vi "PITerm.vi"(0 "System no.":i32=1 min=1 max=4 step=1, 1 "String to Send":string) -> (14 "Comm Window":string)   [LabVIEW 2014]
doc: "Simple Terminal Application.\n\nThis vi can be executed in parallel to any existing PI LabVIEW application. \nPlease run XXX_Configuration_Setup.vi and adjust the System no. on the frontpanel to communicate with your PI device.\n\nShorcut keys:\nReturn: Send\nF5: ERR? (with error translation)\nF12: Additional receive function\nPage Up: History up\nPage down: History down"
panel:
  in  "F5":bool
  in  "Command History":string[](array[string])
  in  "Receive":bool
  out "History length":i32
  in  "History DOWN":bool
  in  "History Index":i32
  in  "History UP":bool
  in  "Send":bool
  in  "Clear":bool
  in  "stop":bool
  # "PITerminal"
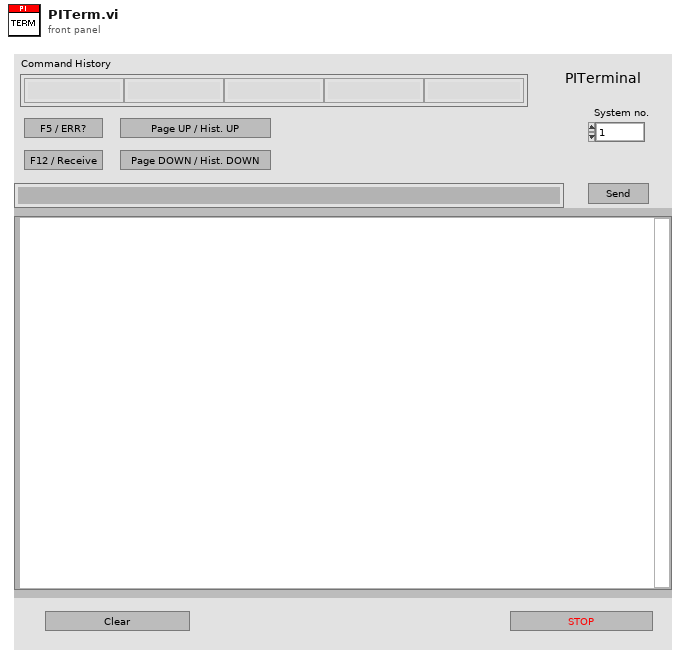
[diagram p1: front panel]
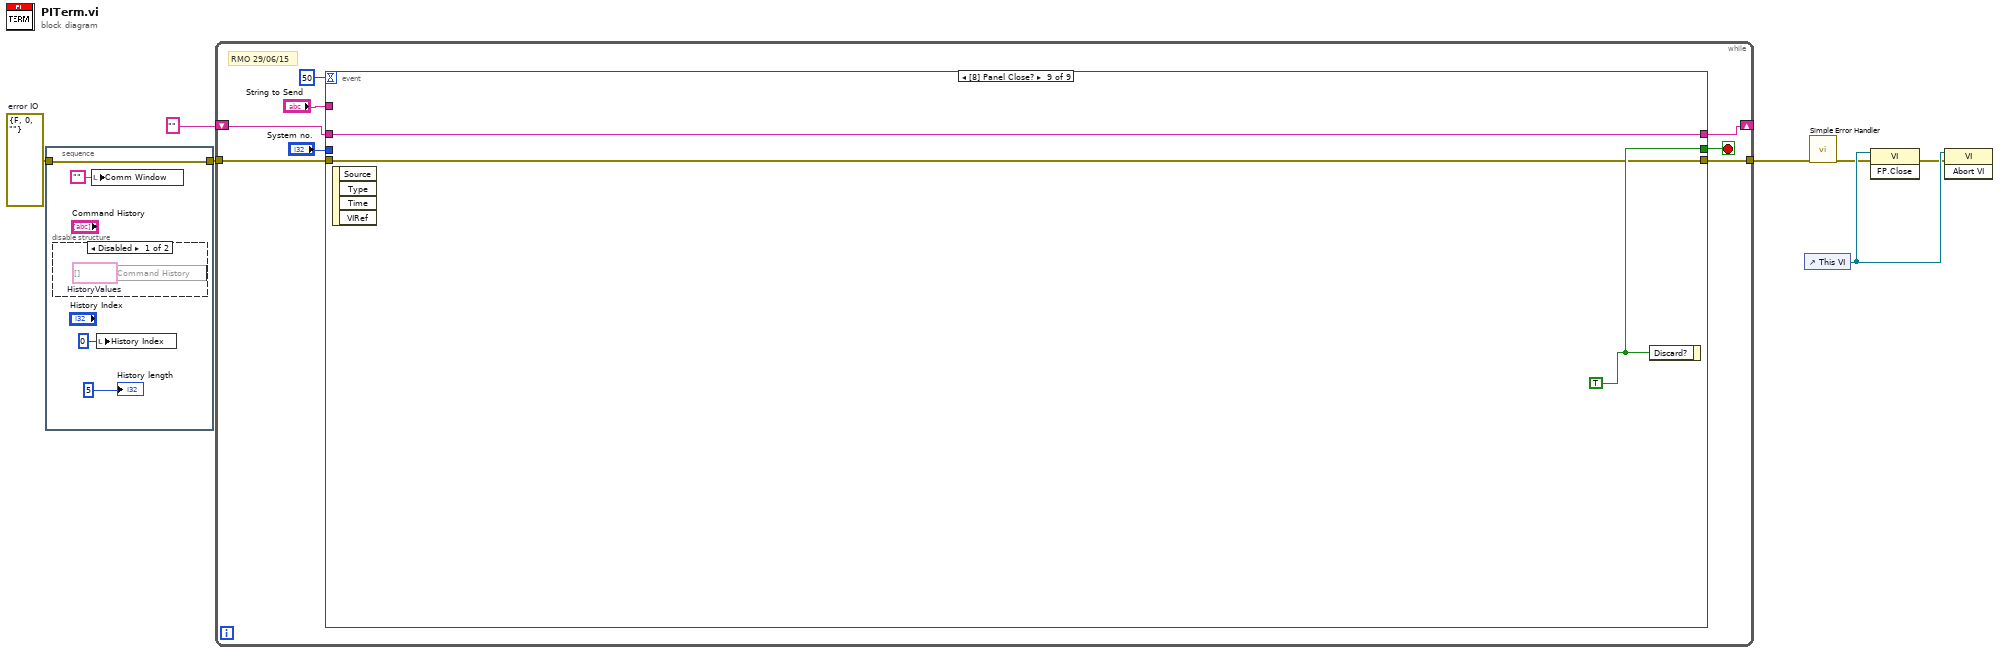
[diagram p0: block diagram]
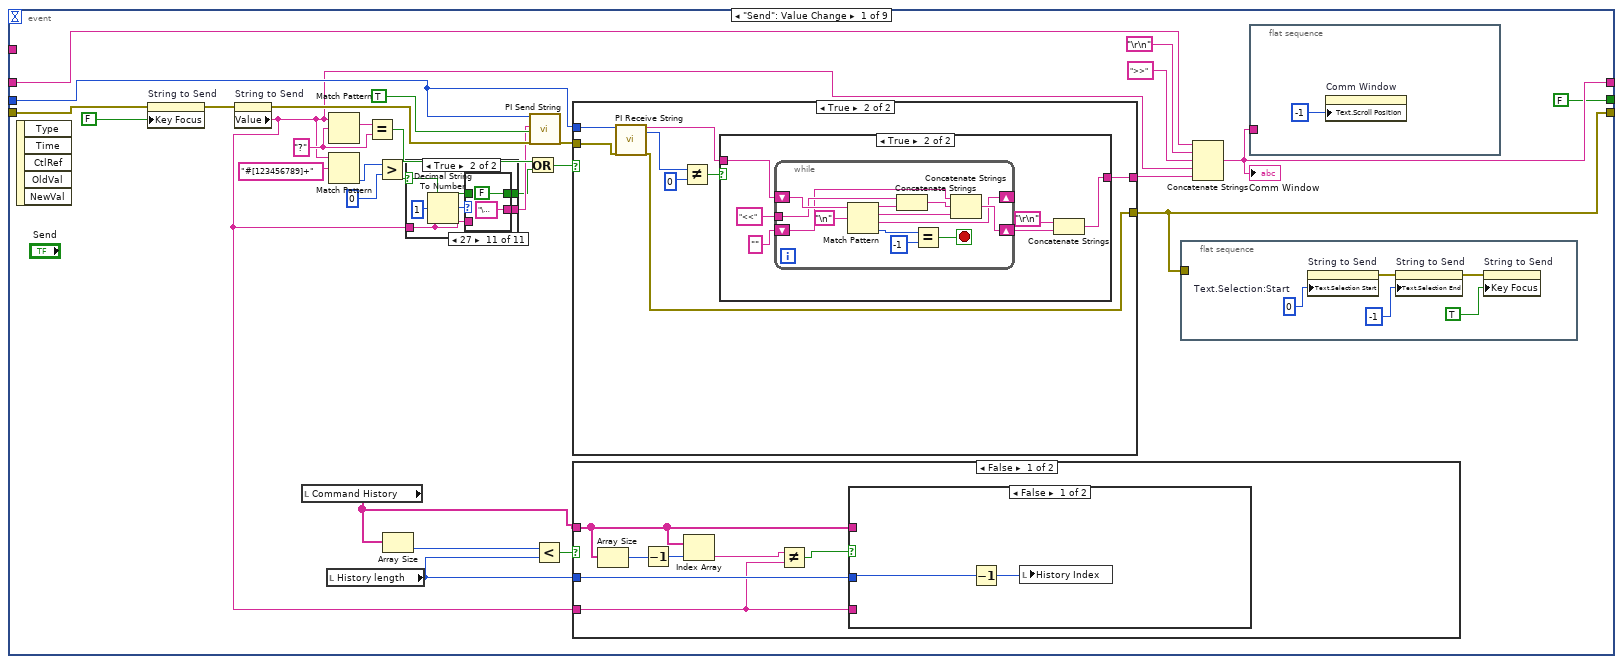
[diagram p3: hidden frame]
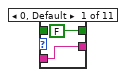
[diagram p5: hidden frame]
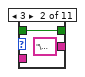
[diagram p6: hidden frame]
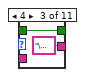
[diagram p7: hidden frame]
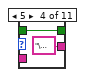
[diagram p8: hidden frame]
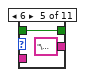
[diagram p9: hidden frame]
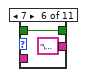
[diagram p10: hidden frame]
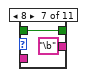
[diagram p11: hidden frame]
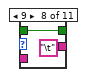
[diagram p12: hidden frame]
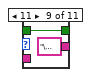
[diagram p13: hidden frame]
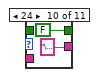
[diagram p14: hidden frame]
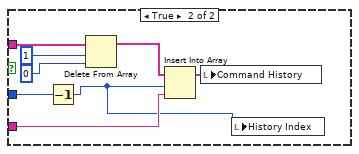
[diagram p15: hidden frame]
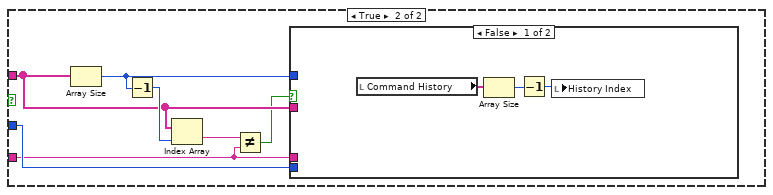
[diagram p16: hidden frame]
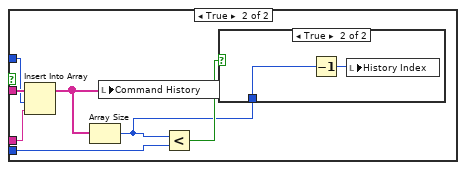
[diagram p17: hidden frame]
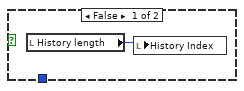
[diagram p18: hidden frame]
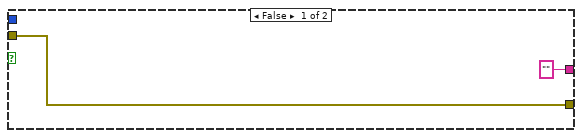
[diagram p19: hidden frame]
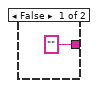
[diagram p20: hidden frame]
diagram:
  w6 = errorcluster {"status"=FALSE, "code"=0, "source"=""}  # error IO
  n1 = stacked-sequence {
    tunnel: w6 -> [w10]
    tunnel: [w10] -> w5
    frame #0 {
      n2 = disable-structure shown="Disabled" {
        frame Disabled {
          w12 = string[] []  # HistoryValues
          n3 = local write "Command History"(w12) -> ()
        }
        frame Enabled {
        }
      }
      n4 = local write "Comm Window"("") -> ()
      n5 = local write "History Index"(0) -> ()
      "History length" <- 5
    }
  }
  n6 = while {
    tunnel: [w19] -> w4
    tunnel: w5 -> [w17]
    shift-right: [w16] -> _
    shift-left: "" -> [w13]
    stop <- w15 stop-if-true
    # "RMO 29/06/15"
    n7 = event shown="[8] Panel Close?" {
      selector: _ -> [_ _ _ _ _ _ _ _ _]
      dyn-events: _ -> [_ _ _ _ _ _ _ _ _]
      timeout: 50 -> [_ _ _ _ _ _ _ _ _]
      tunnel: "String to Send" -> [_ _ _ _ _ _ _ _ _]
      tunnel: [w37 w154 w201 w223 w232 w254 w261 w264 w266] -> w16
      tunnel: [w22 w152 w196 w217 w227 w250 w260 w263 w265] -> w19
      tunnel: "System no." -> [w48 w156 w198 _ _ _ _ _ _]
      tunnel: w17 -> [w36 w157 w199 w216 w227 w250 w260 w263 w265]
      tunnel: [FALSE FALSE FALSE FALSE FALSE FALSE FALSE "stop" w267] -> w15
      tunnel: w13 -> [w47 w155 w200 _ w232 w254 w261 w264 w266]
      event "Send": Value Change {
        w40 = "?"
        n8 = event-data() -> ()  [unwired: 6 out]
        n9 = property on="String to Send" class="Str"(error in=w36, "Key Focus"=FALSE) -> (error out=w34:errorcluster)  [unwired: 1 in, 1 out]
        n10 = property on="String to Send" class="Str"(error in=w34) -> (error out=w33:errorcluster, "Value"=w26:string)  [unwired: 1 in, 1 out]
        n11 = local read "Command History"() -> (w30:string[])
        n12 = local read "History length"() -> (w29:i32)
        n13 = Match Pattern(string=w26, regular expression=w40) -> (match substring=w42:string)  [unwired: 4 out]
        n14 = Match Pattern(string=w26, regular expression="#[123456789]+") -> (offset past match=w28:i32)  [unwired: 4 out]
        n15 = Equal?(x=w42, y=w40) -> (x = y?=w39:bool)
        n16 = Greater?(x=w28, y=0) -> (0:w24:bool)
        n17 = Array Size(array=w30) -> (size(s)=w32:i32)
        n18 = case shown="True" w24 {
          selector: w24 -> [w55 w58]
          tunnel: w26 -> [w56 w59]
          tunnel: [w56 w60] -> w25
          tunnel: [w55 w57] -> w21
          frame False {
          }
          frame True {
            n19 = Decimal String To Number(string=w59, offset=1) -> (number=w61:i32)  [unwired: 2 out]
            n20 = case shown="27" w61 {
              tunnel: [w64 "\u0003" "\u0004" "\u0005" "\u0006" "\u0007" "\b" "\t" "\u000b" "\u0018" "\u001b"] -> w60
              tunnel: w59 -> [w64 _ _ _ _ _ _ _ _ _ _]
              tunnel: w58 -> [_ w65 w67 w69 w71 w73 w75 w77 w79 _ _]
              tunnel: [FALSE w65 w67 w69 w71 w73 w75 w77 w79 FALSE FALSE] -> w57
              frame 0, Default {
              }
              frame 3 {
              }
              frame 4 {
              }
              frame 5 {
              }
              frame 6 {
              }
              frame 7 {
              }
              frame 8 {
              }
              frame 9 {
              }
              frame 11 {
              }
              frame 24 {
              }
              frame 27 {
              }
            }
          }
        }
        n21 = Or(x=w39, y=w21) -> (x .or. y?=w38:bool)
        n22 = call "PI Send String.vi"("System no."=w48, "String to send"=w25, "Attach termination char.?"=TRUE ("Attach Linefeed?"), "error in"=w33) -> ("error out"=w49:errorcluster)  [unwired: 15 out]
        n23 = Less?(x=w32, y=w29) -> (x < y?=w31:bool)
        n24 = case shown="True" w38 {
          tunnel: w49 -> [w124 w132]
          tunnel: [w124 w125] -> w22
          tunnel: w48 -> [_ w131]
          tunnel: ["" w126] -> w43
          frame False {
          }
          frame True {
            n25 = call "PI Receive String.vi"("System no."=w131, "error in"=w132) -> ("String read"=w130:string, "bytes read"=w129:u16, "error out"=w125:errorcluster)  [unwired: 1 in, 14 out]
            n26 = Not Equal?(x=w129, y=u16 0) -> (x != y?=w128:bool)
            n27 = case shown="True" w128 {
              tunnel: w130 -> [_ w139]
              tunnel: ["" w134] -> w126
              frame False {
              }
              frame True {
                n28 = while {
                  tunnel: "<<" -> [w146]
                  shift-right: [w144] -> w135
                  shift-left: "" -> [w142]
                  shift-right: [w143] -> _
                  shift-left: w139 -> [w151]
                  stop <- w147 stop-if-true
                  n29 = Match Pattern(string=w151, regular expression="\n") -> (before substring=w145:string, match substring=w140:string, after substring=w143:string, offset past match=w149:i32)  [unwired: 1 out]
                  n30 = Concatenate Strings(w146, w145) -> (w141:string)
                  n31 = Equal?(x=w149, y=-1) -> (x = y?=w147:bool)
                  n32 = Concatenate Strings(w142, w141, w140) -> (w144:string)
                }
                n33 = Concatenate Strings("\r\n", w135) -> (w134:string)
              }
            }
          }
        }
        n34 = case shown="False" w31 {
          tunnel: w26 -> [w86 w103]
          tunnel: w30 -> [w90 w105]
          tunnel: w29 -> [w91 w108]
          frame False {
            n35 = Array Size(array=w90) -> (size(s)=w88:i32)
            n36 = Decrement(x=w88) -> (x-1=w89:i32)
            n37 = Index Array(array=w90, index=w89) -> (element=w87:string)
            n38 = Not Equal?(x=w87, y=w86) -> (x != y?=w85:bool)
            n39 = case shown="False" w85 {
              tunnel: w90 -> [_ w101]
              tunnel: w86 -> [_ w98]
              tunnel: w91 -> [w93 w95]
              frame False {
                n40 = Decrement(x=w93) -> (x-1=w92:i32)
                n41 = local write "History Index"(w92) -> ()
              }
              frame True {
                n42 = Decrement(x=w95) -> (x-1=w94:i32)
                n43 = Delete From Array(array=w101, length=1, index=0) -> (array with subset deleted=w99:string[])  [unwired: 1 out]
                n44 = Insert Into Array(array=w99, index=w94, new element=w98) -> (w97:string[])
                n45 = local write "Command History"(w97) -> ()
                n46 = local write "History Index"(w94) -> ()
              }
            }
          }
          frame True {
            n47 = Array Size(array=w105) -> (size(s)=w107:i32)
            n48 = Decrement(x=w107) -> (x-1=w106:i32)
            n49 = Index Array(array=w105, index=w106) -> (element=w104:string)
            n50 = Not Equal?(x=w104, y=w103) -> (x != y?=w102:bool)
            n51 = case shown="False" w102 {
              tunnel: w105 -> [_ w118]
              tunnel: w103 -> [_ w117]
              tunnel: w107 -> [_ w116]
              tunnel: w108 -> [_ w114]
              frame False {
                n52 = local read "Command History"() -> (w111:string[])
                n53 = Array Size(array=w111) -> (size(s)=w110:i32)
                n54 = Decrement(x=w110) -> (x-1=w109:i32)
                n55 = local write "History Index"(w109) -> ()
              }
              frame True {
                n56 = Insert Into Array(array=w118, index=w116, new element=w117) -> (w115:string[])
                n57 = Array Size(array=w115) -> (size(s)=w112:i32)
                n58 = local write "Command History"(w115) -> ()
                n59 = Less?(x=w112, y=w114) -> (x < y?=w113:bool)
                n60 = case shown="True" w113 {
                  tunnel: w112 -> [_ w120]
                  frame False {
                    n61 = local read "History length"() -> (w119:i32)
                    n62 = local write "History Index"(w119) -> ()
                  }
                  frame True {
                    n63 = Decrement(x=w120) -> (x-1=w121:i32)
                    n64 = local write "History Index"(w121) -> ()
                  }
                }
              }
            }
          }
        }
        n65 = flat-sequence {
          tunnel: w22 -> [_]
          frame #0 {
            w53 = u32 0  # Text.Selection:Start
            n66 = property on="String to Send" class="Str"("Text.Selection Start"=w53) -> (error out=w52:errorcluster)  [unwired: 2 in, 1 out]
            n67 = property on="String to Send" class="Str"(error in=w52, "Text.Selection End"=-1) -> (error out=w51:errorcluster)  [unwired: 1 in, 1 out]
            n68 = property on="String to Send" class="Str"(error in=w51, "Key Focus"=TRUE) -> ()  [unwired: 1 in, 2 out]
          }
        }
        n69 = Concatenate Strings(w47, "\r\n", ">>", w26, w43) -> (w37:string)
        "Comm Window" <- w37
        n70 = flat-sequence {
          tunnel: w37 -> [_]
          frame #0 {
            n71 = property on="Comm Window" class="Str"("Text.Scroll Position"=-1) -> ()  [unwired: 2 in, 2 out]
          }
        }
      }
      event "Receive": Value Change {
        n72 = event-data() -> ()  [unwired: 7 out]
        n73 = call "PI Receive String.vi"("System no."=w156, "error in"=w157) -> ("String read"=w161:string, "bytes read"=w160:u16, "error out"=w152:errorcluster)  [unwired: 1 in, 14 out]
        n74 = Not Equal?(x=w160, y=u16 0) -> (x != y?=w159:bool)
        n75 = case shown="True" w159 {
          tunnel: w161 -> [_ w174]
          tunnel: ["" w169] -> w162
          frame False {
          }
          frame True {
            n76 = while {
              tunnel: "<<" -> [w181]
              shift-right: [w179] -> w170
              shift-left: "" -> [w177]
              shift-right: [w178] -> _
              shift-left: w174 -> [w186]
              stop <- w182 stop-if-true
              n77 = Match Pattern(string=w186, regular expression="\n") -> (before substring=w180:string, match substring=w175:string, after substring=w178:string, offset past match=w184:i32)  [unwired: 1 out]
              n78 = Concatenate Strings(w181, w180) -> (w176:string)
              n79 = Equal?(x=w184, y=-1) -> (x = y?=w182:bool)
              n80 = Concatenate Strings(w177, w176, w175) -> (w179:string)
            }
            n81 = Concatenate Strings("\r\n", w170) -> (w169:string)
          }
        }
        n82 = Concatenate Strings(w155, w162) -> (w154:string)
        n83 = flat-sequence {
          tunnel: w152 -> [_]
          frame #0 {
            w166 = u32 0  # Text.Selection:Start
            n84 = property on="String to Send" class="Str"("Text.Selection Start"=w166) -> (error out=w165:errorcluster)  [unwired: 2 in, 1 out]
            n85 = property on="String to Send" class="Str"(error in=w165, "Text.Selection End"=-1) -> (error out=w164:errorcluster)  [unwired: 1 in, 1 out]
            n86 = property on="String to Send" class="Str"(error in=w164, "Key Focus"=TRUE) -> ()  [unwired: 1 in, 2 out]
          }
        }
        n87 = flat-sequence {
          tunnel: w154 -> [_]
          frame #0 {
            n88 = property on="Comm Window" class="Str"("Text.Scroll Position"=-1) -> ()  [unwired: 2 in, 2 out]
          }
        }
        n89 = local write "Comm Window"(w154) -> ()
      }
      event "F5": Value Change {
        n90 = event-data() -> ()  [unwired: 7 out]
        n91 = call "ERR?.vi"("System no."=w198, "error in"=w199) -> ("error out"=w191:errorcluster)  [unwired: 17 out]
        n92 = Unbundle By Name(w191) -> ("code"=w189:i32)
        n93 = call "GCSTranslateError.vi"("error in"=w191) -> ("Error Description"=w192:string, "error out"=w197:errorcluster)  [unwired: 17 out]
        n94 = Equal?(x=w189, y=0) -> (x = y?=w194:bool)
        n95 = case shown="False" w194 {
          tunnel: w192 -> [w206 _]
          tunnel: [w211 "<<0  -  (error 0 - \"No error\")"] -> w193
          tunnel: w189 -> [w210 _]
          frame False {
            n96 = Number To Decimal String(number=w210) -> (decimal integer string=w208:string)  [unwired: 1 out]
            n97 = Concatenate Strings("<<", w208, "  -  (error ", w208, " - \"", w206, "\")") -> (w211:string)
          }
          frame True {
          }
        }
        n98 = Concatenate Strings(w200, "\r\n", ">>", "ERR?", "\r\n", w193) -> (w201:string)
        n99 = call <vilib>:"Clear Errors.vi"("error in (no error)"=w197) -> ("error out"=w196:errorcluster)  [unwired: 1 in, 5 out]
        n100 = flat-sequence {
          tunnel: w201 -> [_]
          frame #0 {
            n101 = property on="Comm Window" class="Str"("Text.Scroll Position"=-1) -> ()  [unwired: 2 in, 2 out]
          }
        }
        n102 = local write "Comm Window"(w201) -> ()
      }
      event "Clear": Value Change {
        w221 = u32 0  # Text.Selection:Start
        w223 = ""
        n103 = event-data() -> ()  [unwired: 7 out]
        n104 = property on="String to Send" class="Str"(error in=w216, "Text.Selection Start"=w221) -> (error out=w219:errorcluster)  [unwired: 1 in, 1 out]
        n105 = property on="String to Send" class="Str"(error in=w219, "Text.Selection End"=-1) -> (error out=w218:errorcluster)  [unwired: 1 in, 1 out]
        n106 = local write "Comm Window"(w223) -> ()
        n107 = property on="String to Send" class="Str"(error in=w218, "Key Focus"=TRUE) -> (error out=w217:errorcluster)  [unwired: 1 in, 1 out]
      }
      event "History UP": Value Change {
        n108 = event-data() -> ()  [unwired: 7 out]
        n109 = local read "Command History"() -> (w226:string[])
        n110 = local read "History Index"() -> (w231:i32)
        n111 = Less?(x=w231, y=1) -> (x < y?=w229:bool)
        n112 = case shown="False" w229 {
          tunnel: [w238 0] -> w225
          tunnel: w231 -> [w236 _]
          tunnel: w226 -> [w237 _]
          frame False {
            n113 = Index Array(array=w237, index=w236) -> (element=w235:string)
            n114 = Not Equal?(x=w235, y="") -> (x != y?=w233:bool)
            n115 = case shown="False" w233 {
              tunnel: [w239 w243] -> w238
              tunnel: w236 -> [w241 w242]
              frame False {
                n116 = Decrement(x=w241) -> (x-1=w240:i32)
                n117 = Decrement(x=w240) -> (x-1=w239:i32)
              }
              frame True {
                n118 = Decrement(x=w242) -> (x-1=w243:i32)
              }
            }
          }
          frame True {
          }
        }
        n119 = local write "History Index"(w225) -> ()
        n120 = Index Array(array=w226, index=w225) -> (element=w228:string)
        n121 = local write "String to Send"(w228) -> ()
      }
      event "History DOWN": Value Change {
        n122 = event-data() -> ()  [unwired: 7 out]
        n123 = local read "Command History"() -> (w249:string[])
        n124 = Array Size(array=w249) -> (size(s)=w248:i32)
        n125 = Decrement(x=w248) -> (x-1=w246:i32)
        n126 = local read "History Index"() -> (w253:i32)
        n127 = Decrement(x=w246) -> (x-1=w247:i32)
        n128 = Greater?(x=w253, y=w247) -> (0:w252:bool)
        n129 = case shown="True" w252 {
          tunnel: [w257 w258] -> w255
          tunnel: w253 -> [w256 _]
          tunnel: w246 -> [_ w258]
          frame False {
            n130 = Increment(x=w256) -> (x+1=w257:i32)
          }
          frame True {
          }
        }
        n131 = local write "History Index"(w255) -> ()
        n132 = Index Array(array=w249, index=w255) -> (element=w251:string)
        n133 = local write "String to Send"(w251) -> ()
      }
      event Timeout {
        n134 = event-data() -> ()  [unwired: 4 out]
      }
      event "stop": Value Change {
        n135 = event-data() -> ()  [unwired: 4 out]
      }
      event Panel Close? {
        w267 = TRUE
        n136 = event-data() -> ()  [unwired: 5 out]
        n137 = event-data("Discard?"=w267) -> ()  [unwired: 1 in, 1 out]
      }
    }
  }
  n138 = control-ref of="This VI"() -> (w3:refnum<vi>)
  n139 = call <vilib>:"Simple Error Handler.vi"("error in (no error)"=w4) -> ("error out"=w2:errorcluster)  [unwired: 1 in, 7 out]
  n140 = invoke class="VI" method="FP.Close"(reference=w3, error in=w2) -> (error out=w1:errorcluster)  [unwired: 1 in, 2 out]
  n141 = invoke class="VI" method="Abort VI"(reference=w3, error in=w1) -> ()  [unwired: 1 in, 3 out]
